vi "wa32 ConnectNamedPipe.vi"(8 "error in":errorcluster, 11 "handle":i32) -> (0 "error out":errorcluster, 3 "handle out":i32)   [LabVIEW 2020, in "GOLPI library.lvlib"]
doc: "WinAPI ConnectNamedPipe() wrapper."
uses:
  <vilib>/Utility/error.llb/Error Cluster From Error Code.vi
  <vilib>/ErrorRing/Error Ring.xnode
  GOLPI library.lvlib
  kernel32.dll
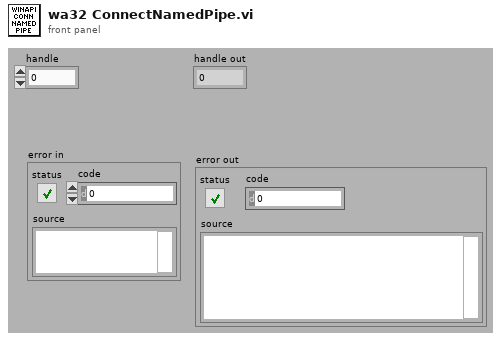
[diagram p1: front panel]
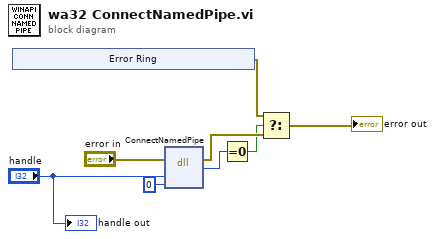
[diagram p0: block diagram]
diagram:
  n1 = xnode "Error Ring"() -> ("error out"=w5:errorcluster)
  n2 = dll-call lib="kernel32.dll" fn="ConnectNamedPipe"(error in="error in", "handle"="handle", "overlapped"=0) -> (error out=w7:errorcluster, "errout"=w4:i32)  [unwired: 4 in, 1 out]
  n3 = Equal To 0?(x=w4) -> (x = 0?=w3:bool)
  n4 = Select(t=w5, s=w3, f=w7) -> (s? t:f=→"error out":errorcluster)
  "handle out" <- "handle"
